vi "Create 2 Hidden Layers.vi"(0 "1st Hidden Layer Neurons":u32, 1 "Output Layer Linear":bool, 2 "Add Bias Inputs":bool=TRUE, 5 "2nd Hidden Layer Neurons":u32, 11 "Error In":errorcluster, 12 "# Inputs":u32, 13 "Output Neurons/Outputs":u32) -> (4 "Neural Network":T1={"Weigths"=[], "Last Layer Linear"=TRUE, "Add Bias Inputs"=TRUE, "# Inputs"=0, "# Output Neurons/Outputs"=0, "Inputs Scaling"={"X Scaling Vector"=[], "Y Scaling Vector"=[]}, "Outputs Scaling"={"X Scaling Vector"=[], "Y Scaling Vector"=[]}}, 15 "Error Out":errorcluster)   [LabVIEW 2013, in "Super Simple Neural Network.lvlib"]
doc: "This VI creates a neural network with 2 hidden layers. This means that the network has 3 layers: input, hidden1, hidden2 and output. Networks implement scaling of input and output values to the range of 0.2 to 0.8. This makes the unipolar sigmoidal activation function of the neurons most effective.\n\n<b> Add Bias Inputs</b> - this setting adds bias inputs of 1 to all neurons of all layers. This greatly imroves the performance of the teaching algorithm.s\n\n<b> Output Layer Linear</b> - If the output values that you want to get from the network are not bound by max and min values you should set the output layer to linear. This setting allows the network to output effectivly beyond the range of values that you teach it with."
uses:
  Super Simple Neural Network.lvlib
  Types/Neural Network.ctl
  Types/2D Array.ctl
  Types/Scaling Info.ctl
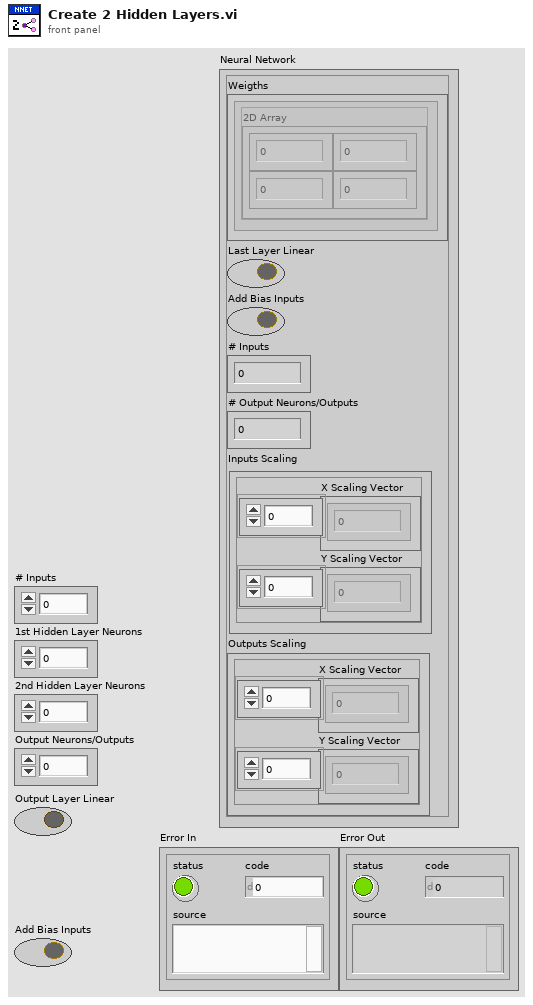
[diagram p1: front panel]
types:
  T1 = typedef "Super Simple Neural Network.lvlib/Neural Network.ctl" = cluster{"Weigths":T2[], "Last Layer Linear":bool, "Add Bias Inputs":bool, "# Inputs":u32, "# Output Neurons/Outputs":u32, "Inputs Scaling":T3, "Outputs Scaling":T3}
  T2 = typedef "Super Simple Neural Network.lvlib/2D Array.ctl" = cluster{"2D Array":dbl[][]}
  T3 = typedef "Super Simple Neural Network.lvlib/Scaling Info.ctl" = cluster{"X Scaling Vector":dbl[], "Y Scaling Vector":dbl[]}
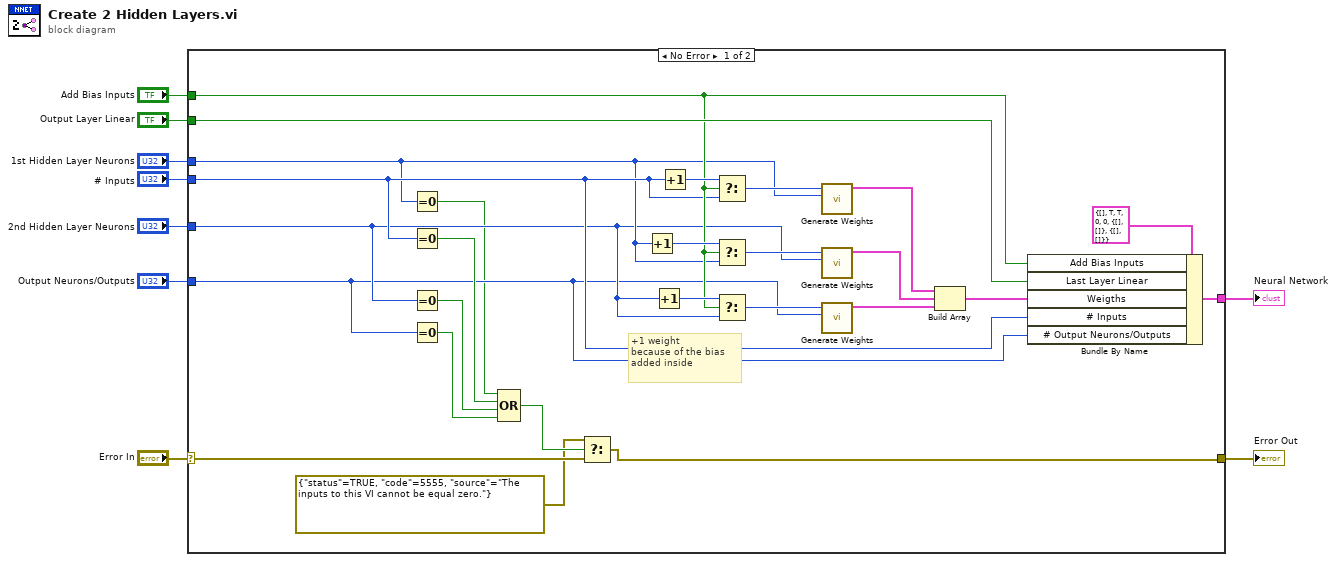
[diagram p0: block diagram]
diagram:
  n1 = case shown="No Error" "Error In" {
    selector: "Error In" -> [w12 w36]
    tunnel: [w35 _] -> w9
    tunnel: "Output Layer Linear" -> [w33 _]
    tunnel: "Add Bias Inputs" -> [w29 _]
    tunnel: "1st Hidden Layer Neurons" -> [w16 _]
    tunnel: "2nd Hidden Layer Neurons" -> [w15 _]
    tunnel: "Output Neurons/Outputs" -> [w14 _]
    tunnel: "# Inputs" -> [w17 _]
    tunnel: [w10 w36] -> w1
    frame No Error {
      # "+1 weight\nbecause of the bias\nadded inside"
      n2 = Equal To 0?(x=w16) -> (x = 0?=w13:bool)
      n3 = Equal To 0?(x=w17) -> (x = 0?=w19:bool)
      n4 = Equal To 0?(x=w15) -> (x = 0?=w20:bool)
      n5 = Equal To 0?(x=w14) -> (x = 0?=w21:bool)
      n6 = Compound Arithmetic op=OR(w13, w19, w20, w21) -> (w18:bool)
      n7 = Select(t=errorcluster {"status"=TRUE, "code"=5555, "source"="The inputs to this VI cannot be equal zero."}, s=w18, f=w12) -> (s? t:f=w10:errorcluster)
      n8 = Increment(x=w16) -> (x+1=w32:u32)
      n9 = Increment(x=w15) -> (x+1=w31:u32)
      n10 = Increment(x=w17) -> (x+1=w30:u32)
      n11 = Select(t=w30, s=w29, f=w17) -> (s? t:f=w27:u32)
      n12 = Select(t=w32, s=w29, f=w16) -> (s? t:f=w25:u32)
      n13 = Select(t=w31, s=w29, f=w15) -> (s? t:f=w23:u32)
      n14 = call "Generate Weights.vi"("Neurons"=w16, "Inputs"=w27) -> ("Layer Weights"=w26:T2)  [unwired: 9 in]
      n15 = call "Generate Weights.vi"("Neurons"=w15, "Inputs"=w25) -> ("Layer Weights"=w24:T2)  [unwired: 9 in]
      n16 = call "Generate Weights.vi"("Neurons"=w14, "Inputs"=w23) -> ("Layer Weights"=w22:T2)  [unwired: 9 in]
      n17 = Build Array(w26, w24, w22) -> (w28:T2[])
      n18 = Bundle By Name(cluster=T1 {"Weigths"=[], "Last Layer Linear"=TRUE, "Add Bias Inputs"=TRUE, "# Inputs"=0, "# Output Neurons/Outputs"=0, "Inputs Scaling"={"X Scaling Vector"=[], "Y Scaling Vector"=[]}, "Outputs Scaling"={"X Scaling Vector"=[], "Y Scaling Vector"=[]}} ("Neural Network"), "Add Bias Inputs"=w29, "Last Layer Linear"=w33, "Weigths"=w28, "# Inputs"=w17, "# Output Neurons/Outputs"=w14) -> (w35:T1)
    }
    frame Error {
    }
  }
  "Neural Network" <- w9
  "Error Out" <- w1
